vi "Encode Image to PNG File Buffer with Alpha.vi"(8 "error in (no error)":errorcluster, 11 "ARGB Image Source in":T1) -> (0 "error out":errorcluster, 3 "Buffer":string)   [LabVIEW 2020, in "image.lvlib"]
doc: "Write an Image file. A broad range of file formats are supported including jpeg, bitmap, png, webp, tiff and others."
uses:
  image.lvlib
  ARGB Image.ctl
  b711c62e-7e14-408f-bb3b-a3086b0dc120.vi
  <vilib>/Utility/error.llb/Error Cluster From Error Code.vi
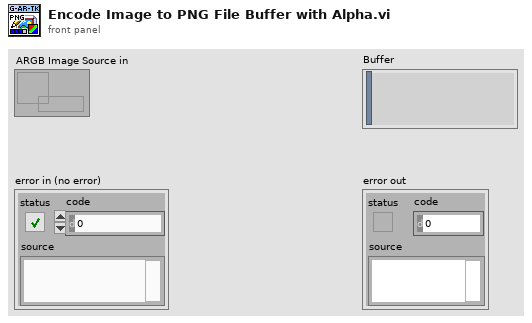
[diagram p1: front panel]
types:
  T1 = typedef "image.lvlib/ARGB Image.ctl" = refnum<data-value>
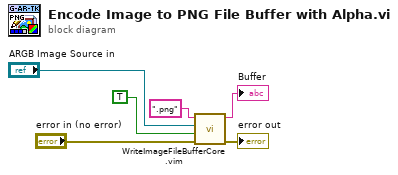
[diagram p0: block diagram]
diagram:
  n1 = call "WriteImageFileBufferCore.vim"("error in (no error)"="error in (no error)", "SaveAlpha"=TRUE, "Src"="ARGB Image Source in", "Extension"=".png") -> ("error out"=→"error out":errorcluster, "Buffer"=→"Buffer":string)  [unwired: 6 in]
